vi "showStimulusOne.vi"(8 "error in (no error)":errorcluster, 10 "index":i32, 11 "Stimulus in":refnum<class "Stimulus.lvclass">) -> (0 "error out":errorcluster, 3 "Stimulus out":refnum<class "Stimulus.lvclass">)   [LabVIEW 2014, in "Stimulus.lvclass"]
uses:
  Stimulus.lvclass
  Stimulus.lvclass/Stimulus.ctl
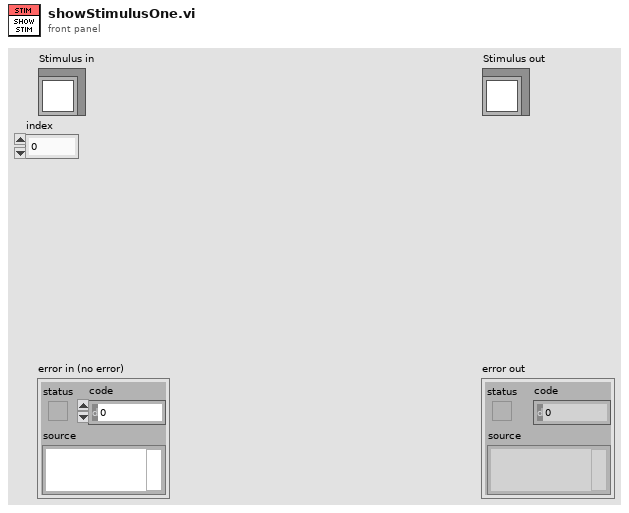
[diagram p1: front panel]
types:
  T1 = typedef "IMAQ Image.ctl" = refnum<image>
  T2 = cluster{"Image":T1, "Window Number (0...15)":i32, "Coordinates (screen)":cluster{"X Position":i32, "Y Position":i32}, "Window name":string, "Time":dbl, "Response \nperiod":dbl, "TI delay":dbl, "Punishment Delay":dbl, "Stim queue":refnum<queue>, "ExpType":enum16{"Orientation", "Calibrate", "Freerun", "BW"}, "Stimuli":string, "Rewarded Stimuli":string, "RI":dbl, "Correct response":bool, "Next Image 2":T1}[]
  T3 = cluster{"Image":T1, "Window Number (0...15)":i32, "Coordinates (screen)":cluster{"X Position":i32, "Y Position":i32}, "Window name":string, "Time":dbl, "Response \nperiod":dbl, "TI delay":dbl, "Punishment Delay":dbl, "Stim queue":refnum<queue>, "ExpType":enum16{"Orientation", "Calibrate", "Freerun", "BW"}, "Stimuli":string, "Rewarded Stimuli":string, "RI":dbl, "Correct response":bool, "Next Image 2":T1}
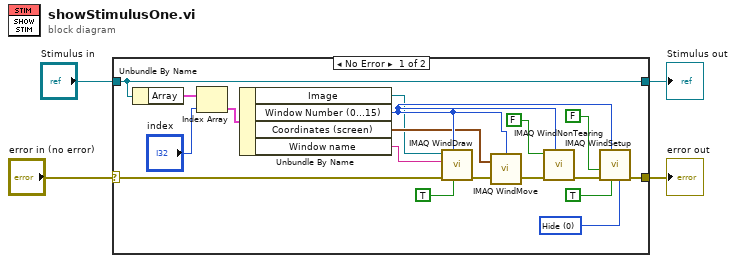
[diagram p0: block diagram]
diagram:
  n1 = case shown="No Error" "error in (no error)" {
    selector: "error in (no error)" -> [w22 w24]
    tunnel: [w21 w24] -> w3
    tunnel: [w6 w23] -> w1
    tunnel: "Stimulus in" -> [w6 w23]
    frame No Error {
      w14 = 0 items=["Hide", "Show", "No change"] ("Scrollbars (No change)")
      n2 = Unbundle By Name(w6) -> ("Array"=w8:T2)
      n3 = Index Array(array=w8, index="index") -> (element=w9:T3)
      n4 = Unbundle By Name(w9) -> ("Image"=w5:T1, "Window Number (0...15)"=w12:i32, "Coordinates (screen)"=w11:cluster{"X Position":i32, "Y Position":i32}, "Window name"=w10:string)
      n5 = call "IMAQ WindDraw"("Resize to Image Size? (Y)"=TRUE, "Window Number (0...15)"=w12, "error in (no error)"=w22, "Title"=w10, "Image"=w5) -> ("error out"=w19:errorcluster)  [unwired: 5 in, 1 out]
      n6 = call "IMAQ WindMove"("Window Number (0...15)"=w12, "Coordinates (screen)"=w11, "error in (no error)"=w19) -> ("error out"=w18:errorcluster)  [unwired: 2 in, 1 out]
      n7 = call "IMAQ WindNonTearing"("Window Number"=w12, "error in (no error)"=w18, "NonTearing? (True)"=FALSE) -> ("error out"=w13:errorcluster)  [unwired: 7 in, 1 out]
      n8 = call "IMAQ WindSetup"("Scrollbars (No change)"=w14, "Window is floating? (No)"=TRUE, "Window Number (0...15)"=w12, "error in (no error)"=w13, "Window has title bar? (Yes)"=FALSE) -> ("error out"=w21:errorcluster)  [unwired: 6 in]
    }
    frame Error {
    }
  }
  "error out" <- w3
  "Stimulus out" <- w1
